vi "Clear Arbitrary Sequence [SEQ].vi"(8 "error in (no error)":errorcluster, 9 "sequence handle (0)":i32, 11 "CS++Fgen in":refnum<class "CS++Fgen.lvclass">) -> (0 "error out":errorcluster, 3 "CS++Fgen out":refnum<class "CS++Fgen.lvclass">)   [LabVIEW 2013, in "CS++Fgen.lvlib" / "CS++Fgen.lvclass"]
doc: "This VI removes a previously created arbitrary sequence from the function generator's memory and invalidates the sequence's handle.\n\nNotes:\n\n(1) This VI is part of the IviFgenArbSeq [SEQ] extension group."
uses:
  CS++Fgen.lvclass
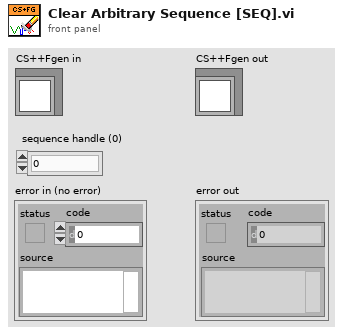
[diagram p1: front panel]
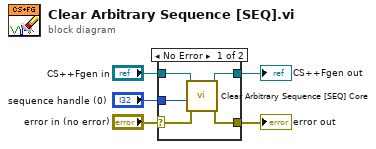
[diagram p0: block diagram]
diagram:
  n1 = case shown="No Error" "error in (no error)" {
    selector: "error in (no error)" -> [w9 w12]
    tunnel: [w8 w12] -> w4
    tunnel: [w6 w11] -> w2
    tunnel: "CS++Fgen in" -> [w7 w11]
    tunnel: "sequence handle (0)" -> [w10 _]
    frame No Error {
      n2 = call-dynamic "Clear Arbitrary Sequence [SEQ] Core.vi"("error in (no error)"=w9, "sequence handle (0)"=w10, "CS++Fgen in"=w7) -> ("error out"=w8:errorcluster, "CS++Fgen out"=w6:refnum<class "CS++Fgen.lvclass">)  [unwired: 7 in]
    }
    frame Error {
    }
  }
  "error out" <- w4
  "CS++Fgen out" <- w2
